vi "输出分辨率计算.vi"(6 "偏移量":sgl, 7 "数值1":dbl, 8 "分辨率":dbl, 9 "数值 4":dbl, 10 "数值 3":dbl, 11 "数值 2":dbl) -> (0 "输出4":dbl, 1 "输出3":dbl, 2 "输出2":dbl, 3 "输出1":dbl)   [LabVIEW 2013]
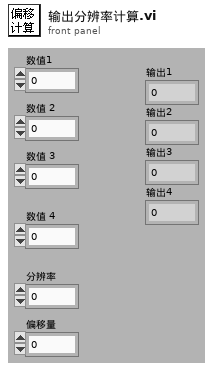
[diagram p1: front panel]
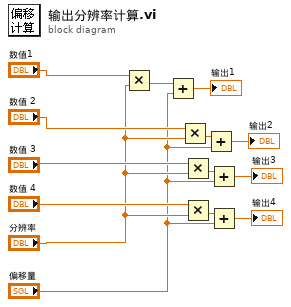
[diagram p0: block diagram]
diagram:
  n1 = Multiply(x="数值1", y="分辨率") -> (x*y=w13:dbl)
  n2 = Add(x=w13, y="偏移量") -> (x+y=→"输出1":dbl)
  n3 = Multiply(x="数值 2", y="分辨率") -> (x*y=w12:dbl)
  n4 = Multiply(x="数值 3", y="分辨率") -> (x*y=w10:dbl)
  n5 = Multiply(x="数值 4", y="分辨率") -> (x*y=w8:dbl)
  n6 = Add(x=w12, y="偏移量") -> (x+y=→"输出2":dbl)
  n7 = Add(x=w10, y="偏移量") -> (x+y=→"输出3":dbl)
  n8 = Add(x=w8, y="偏移量") -> (x+y=→"输出4":dbl)
